vi "Read offsetType.vi"(8 "error in (no error)":errorcluster, 11 "OffsetStatus in":refnum<class "OffsetStatus.lvclass">) -> (0 "error out":errorcluster, 2 "offsetType":T1, 3 "OffsetStatus out":refnum<class "OffsetStatus.lvclass">)   [LabVIEW 2022 SP3, in "TCSDataDefinitions.lvlib" / "TCSPublicStatus.lvlib" / "OffsetStatus.lvclass"]
uses:
  OffsetStatus.lvclass
  TCSCommand/OffsetCommands/OffsetDef/Enumerations/OffsetType.ctl
  OffsetStatus.lvclass/OffsetStatus.ctl
  TCSCommand/OffsetCommands/OffsetCommands.lvlib
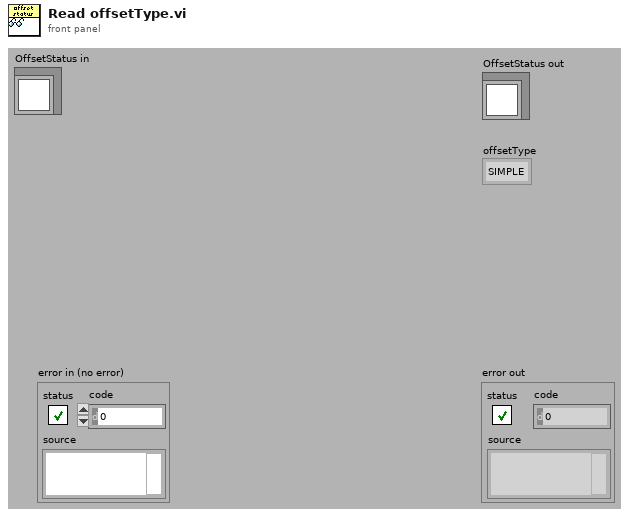
[diagram p1: front panel]
types:
  T1 = typedef "TCSDataDefinitions.lvlib/TCSCommand.lvlib/OffsetCommands.lvlib/OffsetType.ctl" = enum16{"SIMPLE", "TPLANE", "PA"}
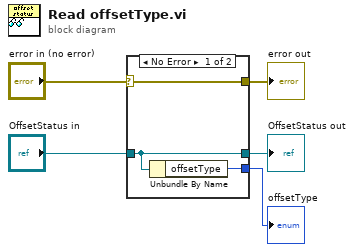
[diagram p0: block diagram]
diagram:
  n1 = case shown="No Error" "error in (no error)" {
    selector: "error in (no error)" -> [w8 w9]
    tunnel: [w8 w9] -> w4
    tunnel: [w7 w10] -> w1
    tunnel: "OffsetStatus in" -> [w7 w10]
    tunnel: [w6 _] -> w3
    frame No Error {
      n2 = Unbundle By Name(w7) -> ("offsetType"=w6:T1)
    }
    frame Error {
    }
  }
  "error out" <- w4
  "offsetType" <- w3
  "OffsetStatus out" <- w1
